vi "getAll.vi"(8 "error in (no error)":errorcluster, 11 "RP100 in":refnum<class "RP100.lvclass">) -> (0 "error out":errorcluster, 2 "getAll":variant, 3 "RP100 out":refnum<class "RP100.lvclass">)   [LabVIEW 2016, in "RP100.lvclass"]
uses:
  RP100.lvclass
  C:/Program Files (x86)/National Instruments/LabVIEW 2016/user.lib/LevyLab/Levylab Instruments/SMOs/Instrument/Instrument.lvclass
  Typedefs/Output Channel--Enum.ctl
  <userlib>/LevyLab/Levylab Instruments/SMOs/Instrument/Instrument.lvclass/Instrument.ctl
  RP100.lvclass/RP100.ctl
  <userlib>/LevyLab/Levylab Instruments/SMOs/Instrument/Instrument.lvclass
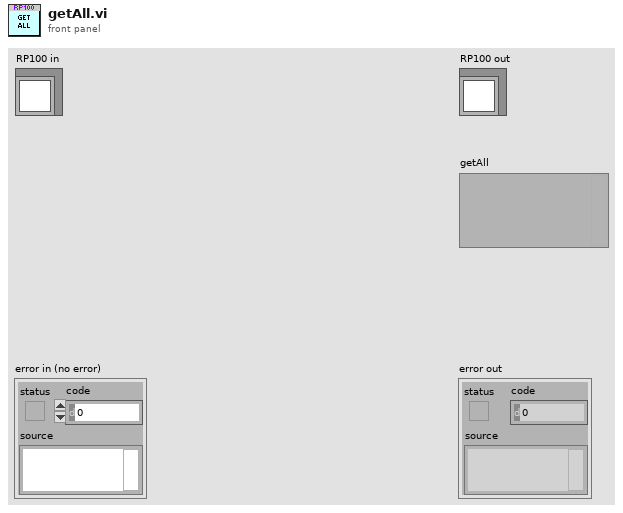
[diagram p1: front panel]
types:
  T1 = typedef "RP100.lvclass/Output Channel--Enum.ctl" = enum16{"Output 1", "Output 2"}
  T2 = typedef "RP100.lvclass/Output State--Enum.ctl" = enum16{"Shorted", "Enabled"}
  T3 = typedef "RP100.lvclass/getAll.ctl" = cluster{"Output State Ch1":string, "Output State Ch2":string, "Level (V) Ch1":dbl, "Level (V) Ch2":dbl, "Slew (V/s) Ch1":dbl, "Slew (V/s) Ch2":dbl, "measured V Ch1":dbl, "measured V Ch2":dbl, "measured I Ch1":dbl, "measured I Ch2":dbl}
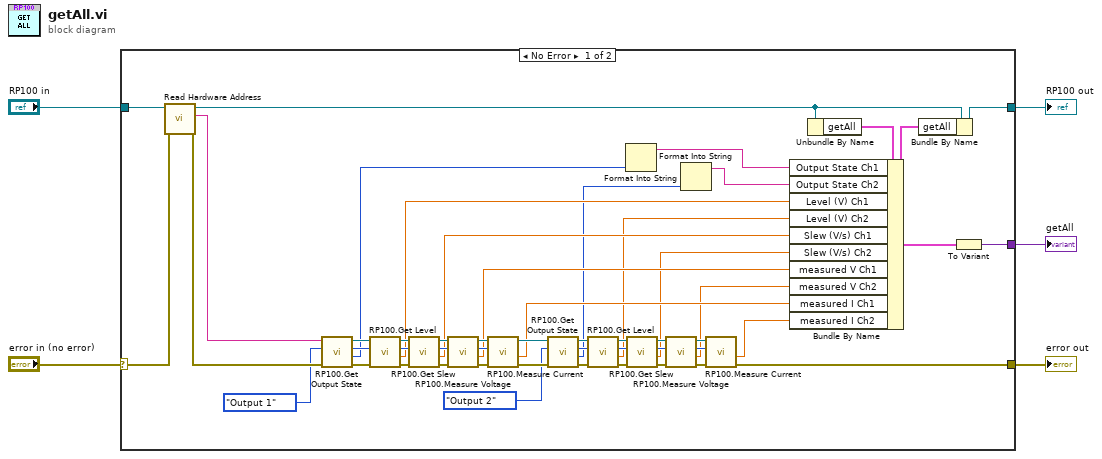
[diagram p0: block diagram]
diagram:
  n1 = case shown="No Error" "error in (no error)" {
    selector: "error in (no error)" -> [w54 w57]
    tunnel: [w29 w57] -> w4
    tunnel: [w12 w56] -> w3
    tunnel: "RP100 in" -> [w55 w56]
    tunnel: [w10 _] -> w1
    frame No Error {
      n2 = call <userlib>:"Read Hardware Address.vi"("error in (no error)"=w54, "Instrument in"=w55) -> ("error out"=w45:errorcluster, "Address"=w44:string, "Instrument out"=w13:refnum<class "RP100.lvclass">)  [unwired: 7 in]
      n3 = call "RP100.Get Output State.vi"("error in (no error)"=w45, "Output Channel"=Output_Channel--Enum."Output 1", "VISA resource name"=w44) -> ("error out"=w40:errorcluster, "Output State"=w9:T2, "Output Channel"=w28:T1, "VISA Refnum out"=w41:refnum<visa-resource-name>)  [unwired: 5 in]
      n4 = call "RP100.Get Level.vi"("error in (no error)"=w40, "Output Channel"=w28, "VISA resource name"=w41) -> ("error out"=w38:errorcluster, "Level (V)"=w22:dbl, "Output Channel"=w27:T1, "VISA Refnum out"=w39:refnum<visa-resource-name>)  [unwired: 5 in]
      n5 = call "RP100.Get Slew.vi"("error in (no error)"=w38, "Output Channel"=w27, "VISA resource name"=w39) -> ("error out"=w36:errorcluster, "Slew (V/s)"=w21:dbl, "Output Channel"=w26:T1, "VISA Refnum out"=w37:refnum<visa-resource-name>)  [unwired: 5 in]
      n6 = call "RP100.Measure Voltage.vi"("error in (no error)"=w36, "Output"=w26, "VISA resource name"=w37) -> ("error out"=w52:errorcluster, "measured V"=w20:dbl, "Output"=w51:T1, "VISA Refnum out"=w53:refnum<visa-resource-name>)  [unwired: 5 in]
      n7 = call "RP100.Measure Current.vi"("error in (no error)"=w52, "Output Channel"=w51, "VISA resource name"=w53) -> ("error out"=w47:errorcluster, "measured I"=w19:dbl, "VISA Refnum out"=w46:refnum<visa-resource-name>)  [unwired: 5 in, 1 out]
      n8 = call "RP100.Get Output State.vi"("error in (no error)"=w47, "Output Channel"=Output_Channel--Enum."Output 2", "VISA resource name"=w46) -> ("error out"=w34:errorcluster, "Output State"=w7:T2, "Output Channel"=w25:T1, "VISA Refnum out"=w35:refnum<visa-resource-name>)  [unwired: 5 in]
      n9 = call "RP100.Get Level.vi"("error in (no error)"=w34, "Output Channel"=w25, "VISA resource name"=w35) -> ("error out"=w32:errorcluster, "Level (V)"=w18:dbl, "Output Channel"=w24:T1, "VISA Refnum out"=w33:refnum<visa-resource-name>)  [unwired: 5 in]
      n10 = Format Into String(w9) -> (resulting string=w8:string)  [unwired: 3 in, 1 out]
      n11 = call "RP100.Get Slew.vi"("error in (no error)"=w32, "Output Channel"=w24, "VISA resource name"=w33) -> ("error out"=w30:errorcluster, "Slew (V/s)"=w17:dbl, "Output Channel"=w23:T1, "VISA Refnum out"=w31:refnum<visa-resource-name>)  [unwired: 5 in]
      n12 = call "RP100.Measure Voltage.vi"("error in (no error)"=w30, "Output"=w23, "VISA resource name"=w31) -> ("error out"=w49:errorcluster, "measured V"=w16:dbl, "Output"=w50:T1, "VISA Refnum out"=w48:refnum<visa-resource-name>)  [unwired: 5 in]
      n13 = Format Into String(w7) -> (resulting string=w6:string)  [unwired: 3 in, 1 out]
      n14 = call "RP100.Measure Current.vi"("error in (no error)"=w49, "Output Channel"=w50, "VISA resource name"=w48) -> ("error out"=w29:errorcluster, "measured I"=w15:dbl)  [unwired: 5 in, 2 out]
      n15 = Unbundle By Name(w13) -> ("getAll"=w14:T3)
      n16 = Bundle By Name(cluster=w14, "Output State Ch1"=w8, "Output State Ch2"=w6, "Level (V) Ch1"=w22, "Level (V) Ch2"=w18, "Slew (V/s) Ch1"=w21, "Slew (V/s) Ch2"=w17, "measured V Ch1"=w20, "measured V Ch2"=w16, "measured I Ch1"=w19, "measured I Ch2"=w15) -> (w11:T3)
      n17 = Bundle By Name(cluster=w13, "getAll"=w11) -> (w12:refnum<class "RP100.lvclass">)
      n18 = To Variant(anything=w11) -> (Variant=w10:variant)
    }
    frame Error {
    }
  }
  "error out" <- w4
  "RP100 out" <- w3
  "getAll" <- w1
